vi "CommonVIs_ListFilesRecursive.vi"(1 "directory path":path, 2 "FileSearchPattern":string, 3 "IgnoreClassMemberVIs(False)":bool, 4 "SearchInLLBs(True)":bool=TRUE, 5 "error in (no error)":errorcluster, 6 "RecusiveSearch(True)":bool=TRUE) -> (15 "dup path":path, 16 "Files":path[](array[path]), 17 "Directories":path[](array[path]), 19 "error out":errorcluster)   [LabVIEW 2020]
doc: "Recursively deletes contents of a directory, including the directory itself as default.\nif <B>deleteTopDirAlso</B> is set to false, the selected directory will not be removed."
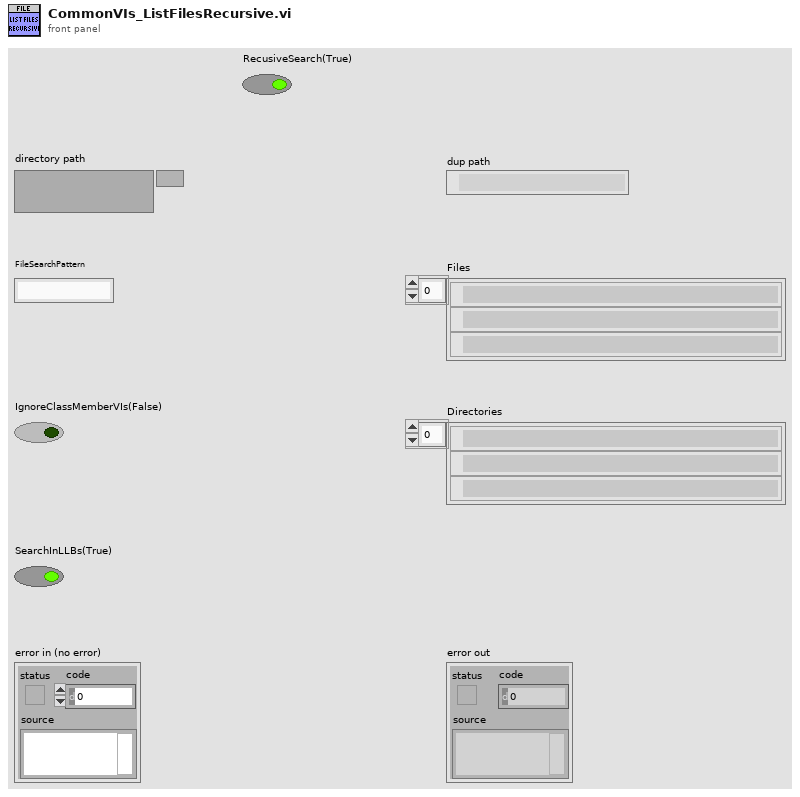
[diagram p1: front panel]
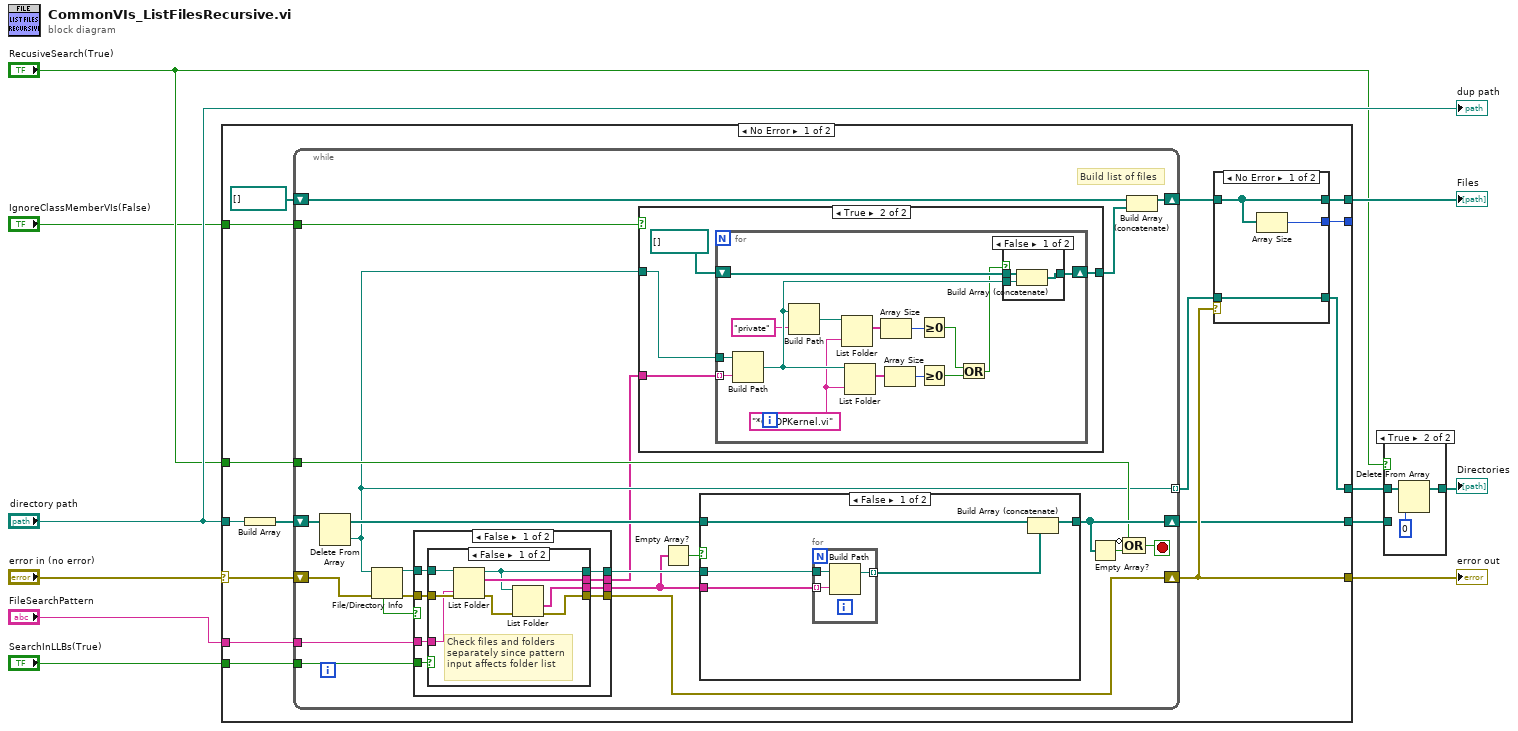
[diagram p0: block diagram]
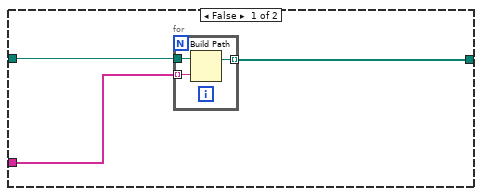
[diagram p4: hidden frame]
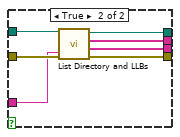
[diagram p7: hidden frame]
diagram:
  n1 = case shown="No Error" "error in (no error)" {
    selector: "error in (no error)" -> [w23 w115]
    tunnel: "directory path" -> [w26 _]
    tunnel: [w16 _] -> w7
    tunnel: [w15 _] -> _
    tunnel: [w20 w115] -> w11
    tunnel: "SearchInLLBs(True)" -> [w22 _]
    tunnel: [w18 _] -> w2
    tunnel: "FileSearchPattern" -> [w21 _]
    tunnel: "RecusiveSearch(True)" -> [w14 _]
    tunnel: [w13 _] -> w1
    tunnel: "IgnoreClassMemberVIs(False)" -> [w12 _]
    frame No Error {
      n2 = Build Array(w26) -> (w25:path[])
      n3 = while {
        shift-left: path[] [] ("Array Constant") -> [w49]
        shift-right: [w51] -> w17
        shift-left: w25 -> [w50]
        shift-right: [w42] -> w13
        shift-right: [w46] -> w20
        shift-left: w23 -> [w39]
        tunnel: w22 -> [w45]
        tunnel: [w32] -> w19 mode=indexing
        tunnel: w21 -> [w44]
        tunnel: w14 -> [w37]
        tunnel: w12 -> [w30]
        stop <- w34 stop-if-true
        # "Build list of files"
        n4 = Delete From Array(array=w50) -> (deleted portion=w32:path, array with subset deleted=w48:path[])  [unwired: 2 in]
        n5 = File/Directory Info(path=w32, error in=w39) -> (path out=w40:path, error out=w41:errorcluster, shortcut=w38:bool)  [unwired: 4 out]
        n6 = case shown="False" w38 {
          tunnel: [w97 _] -> w31
          tunnel: [w96 w114] -> w47
          tunnel: [w95 w113] -> w46
          tunnel: w45 -> [w94 _]
          tunnel: w44 -> [w93 _]
          tunnel: [w92 _] -> w43
          tunnel: w41 -> [w91 w113]
          tunnel: w40 -> [w90 w114]
          frame False {
            n7 = case shown="False" w94 {
              tunnel: [w105 w109] -> w97
              tunnel: [w99 w108] -> w92
              tunnel: w90 -> [w104 w112]
              tunnel: [w98 w110] -> w96
              tunnel: [w100 w107] -> w95
              tunnel: w91 -> [w103 w111]
              tunnel: w93 -> [w102 w106]
              frame False {
                # "Check files and folders\nseparately since pattern\ninput affects folder list"
                n8 = List Folder(path=w104, pattern=w102, error in=w103) -> (path out=w98:path, filenames=w105:string[], error out=w101:errorcluster)  [unwired: 1 in, 1 out]
                n9 = List Folder(path=w98, error in=w101) -> (folder names=w99:string[], error out=w100:errorcluster)  [unwired: 2 in, 2 out]
              }
              frame True {
                n10 = call <vilib>:"List Directory and LLBs.vi"("pattern"=w106, "error in (no error)"=w111, "Folder Path"=w112) -> ("error out"=w107:errorcluster, "Folders and LLBs"=w108:string[], "Files sans LLBs"=w109:string[], "dup Folder Path"=w110:path)  [unwired: 5 in]
              }
            }
          }
          frame True {
            # "Do not attempt to recurse the contents\nof folder shortcuts"
          }
        }
        n11 = case shown="True" w30 {
          tunnel: w32 -> [w54 w59]
          tunnel: [w53 w60] -> w33
          tunnel: w31 -> [w52 w58]
          frame False {
            n12 = for {
              tunnel: w54 -> [w57]
              tunnel: [w56] -> w53 mode=indexing
              tunnel: w52 -> [w55] mode=indexing
              n13 = Build Path(base path=w57, name or relative path=w55) -> (appended path=w56:path)
            }
          }
          frame True {
            n14 = for {
              tunnel: w59 -> [w76]
              tunnel: w58 -> [w75] mode=indexing
              shift-right: [w72] -> w60
              shift-left: path[] [] -> [w73]
              w69 = "*GOOPKernel.vi" ("pattern")
              n15 = Build Path(base path=w76, name or relative path=w75) -> (appended path=w74:path)
              n16 = Build Path(base path=w74, name or relative path="private") -> (appended path=w70:path)
              n17 = List Folder(path=w70, pattern=w69) -> (filenames=w67:string[])  [unwired: 1 in, 4 out]
              n18 = List Folder(path=w74, pattern=w69) -> (filenames=w68:string[])  [unwired: 1 in, 4 out]
              n19 = Array Size(array=w67) -> (size(s)=w65:i32)
              n20 = Array Size(array=w68) -> (size(s)=w66:i32)
              n21 = Greater Or Equal To 0?(x=w65) -> (x >= 0?=w63:bool)
              n22 = Greater Or Equal To 0?(x=w66) -> (x >= 0?=w64:bool)
              n23 = Or(x=w63, y=w64) -> (x .or. y?=w62:bool)
              n24 = case shown="False" w62 {
                tunnel: w73 -> [w79 w80]
                tunnel: [w78 w80] -> w72
                tunnel: w74 -> [w77 _]
                frame False {
                  n25 = Build Array (concatenate)(w79, w77) -> (w78:path[])
                }
                frame True {
                }
              }
            }
          }
        }
        n26 = Empty Array?(array=w43) -> (empty?=w36:bool)
        n27 = case shown="False" w36 {
          tunnel: w48 -> [w83 w89]
          tunnel: [w84 w89] -> w42
          tunnel: w47 -> [w85 _]
          tunnel: w43 -> [w81 _]
          frame False {
            n28 = for {
              tunnel: w85 -> [w88]
              tunnel: [w87] -> w82 mode=indexing
              tunnel: w81 -> [w86] mode=indexing
              n29 = Build Path(base path=w88, name or relative path=w86) -> (appended path=w87:path)
            }
            n30 = Build Array (concatenate)(w83, w82) -> (w84:path[])
          }
          frame True {
          }
        }
        n31 = Empty Array?(array=w42) -> (empty?=w35:bool)
        n32 = Compound Arithmetic op=OR(invert w37, w35) -> (w34:bool)
        n33 = Build Array (concatenate)(w49, w33) -> (w51:path[])
      }
      n34 = case shown="No Error" w20 {
        tunnel: w19 -> [w29 _]
        tunnel: [w29 _] -> w18
        tunnel: w17 -> [w28 _]
        tunnel: [w28 _] -> w16
        tunnel: [w27 _] -> w15
        frame No Error {
          n35 = Array Size(array=w28) -> (size(s)=w27:i32)
        }
        frame Error {
          # "Output empty\narrays if an\nerror occurred\nduring the list"
        }
      }
    }
    frame Error {
    }
  }
  "error out" <- w11
  "Files" <- w7
  n36 = case shown="True" "RecusiveSearch(True)" {
    tunnel: w2 -> [_ w119]
    tunnel: [w116 w117] -> w6
    tunnel: w1 -> [w116 _]
    frame False {
    }
    frame True {
      n37 = Delete From Array(array=w119, index=0) -> (array with subset deleted=w117:path[])  [unwired: 1 in, 1 out]
    }
  }
  "Directories" <- w6
  "dup path" <- "directory path"
